vi "Example-AI Scope IN+Signal Processing+AO Wavegen OUT.vi"() -> ()   [LabVIEW 2018]
uses:
  <vilib>/Analysis/3filter.llb/Filter Passband Type.ctl
  <vilib>/Analysis/NI_AALBase.lvlib
  <vilib>/Analysis/3filter.llb/Butterworth Filter (DBL).vi
panel:
  out "Description":string
  out "SerialNumber":string
  out "return":i32
  in  "timeout":i32=1
  in  "delay(ms)":i32=10
  in  "Getscope":bool
  in  "Filter Config 2":T2={"filter type"=enum."Lowpass", "sampling freq: fs"=800000.0, "high cutoff freq: fh"=10000000.0, "low cutoff freq: fl"=100000.0, "order"=2} {"sampling freq: fs" format="%0.2f"; "high cutoff freq: fh" format="%0.2f"; "low cutoff freq: fl" format="%0.4f"}
  in  "Filter Config":T2={"filter type"=enum."Lowpass", "sampling freq: fs"=800000.0, "high cutoff freq: fh"=10000000.0, "low cutoff freq: fl"=1000.0, "order"=2} {"sampling freq: fs" format="%0.2f"; "high cutoff freq: fh" format="%0.2f"; "low cutoff freq: fl" format="%0.4f"}
  in  "停止":bool
  in  "CH2":T3={"ch"=1, "amp"=1.0, "vOffset"=0.0, "hzFrequency"=2000, "percentageSymmetry"=50.0, "degreePhase"=0.0, "func"=enum."Sine"}
  in  "CH1":T3={"ch"=0, "amp"=1.0, "vOffset"=0.0, "hzFrequency"=2000, "percentageSymmetry"=50.0, "degreePhase"=0.0, "func"=enum."Sine"}
  out "Scope Graph":cluster{"voltages":dbl[], "voltages":dbl[]}[](graph) caption="XY图"
  in  "trigcond":enum16{"Raising", "Falling", "Either"}(ring)
  in  "trigsrc":T4(ring)=enum."DetectorAnalogInCH1"
  in  "trigtype":enum16{"edge", "pulse", "trasition"}(ring)
  in  "enable 2":bool=TRUE
  in  "range 2":dbl=5.0
  in  "voltsLevel":dbl
  in  "range":dbl=5.0
  in  "enable":bool=TRUE
  in  "buffersize":i32=2048
  out "Scope returns":i32[](array[numeric])
  in  "fre":i32=800000
  out "error out":errorcluster caption="错误输出"
  out "ftHandle out":u64=372147880
  in  "Device Index":i32
  # "Scope Config"
  # "Function Wave Generation"
  # "Filter"
  # "Tips: CH1 Filter fl < Wavegen Frequency"
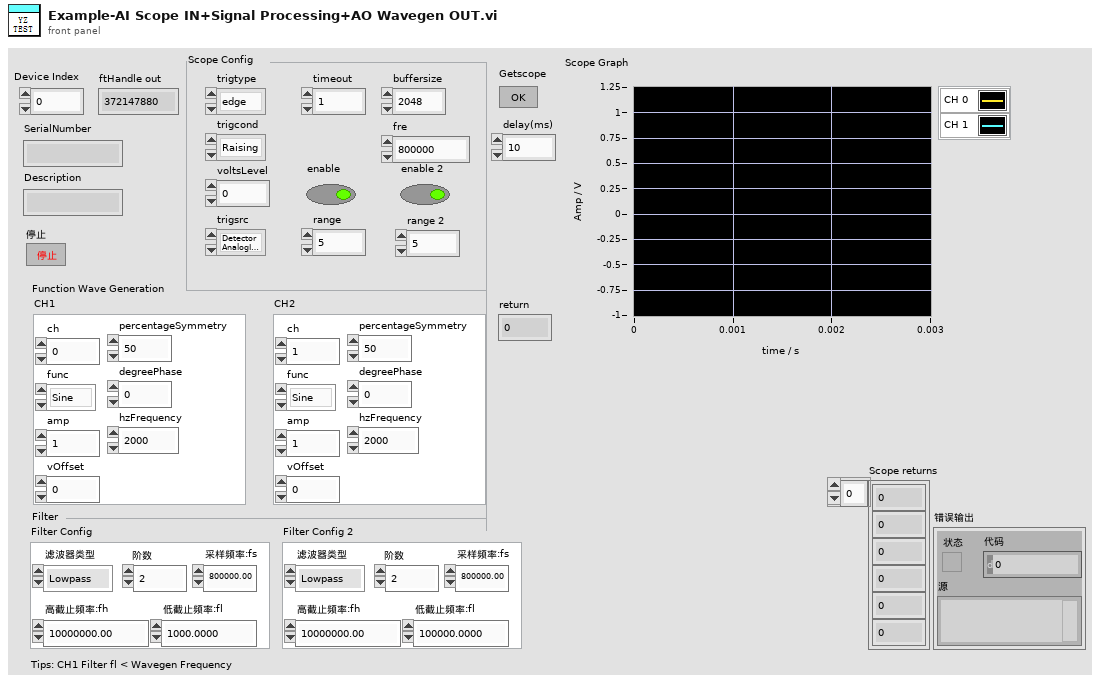
[diagram p1: front panel]
types:
  T1 = typedef "NI_AALBase.lvlib/Filter Passband Type.ctl" = enum32{"Lowpass", "Highpass", "Bandpass", "Bandstop"}
  T2 = cluster{"filter type":T1, "sampling freq: fs":dbl, "high cutoff freq: fh":dbl, "low cutoff freq: fl":dbl, "order":i32}
  T3 = cluster{"ch":i32, "amp":dbl, "vOffset":dbl, "hzFrequency":i32, "percentageSymmetry":dbl, "degreePhase":dbl, "func":enum8{"DC", "Sine", "Square", "Triangle", "RampUp", "RampDown", "Noise", "Pulse", "Trapezium", "SinePower", "Custom", "Play"}}
  T4 = enum16{"None", "DetectorAnalogInCH1", "DetectorAnalogInCH2", "AnalogOut1", "AnalogOut2", "DetectorDigitalIn", "DigitalOut", "Manule", "External 1", "External 2", "DigitalIn"}
  T5 = enum16{"CLIFFStateReady", "CLIFFStateArmed", "CLIFFStateDone", "CLIFFStateRunning", "CLIFFStateConfig", "CLIFFStatePrefill", "CLIFFStateTriggered", "CLIFFStateWait"}
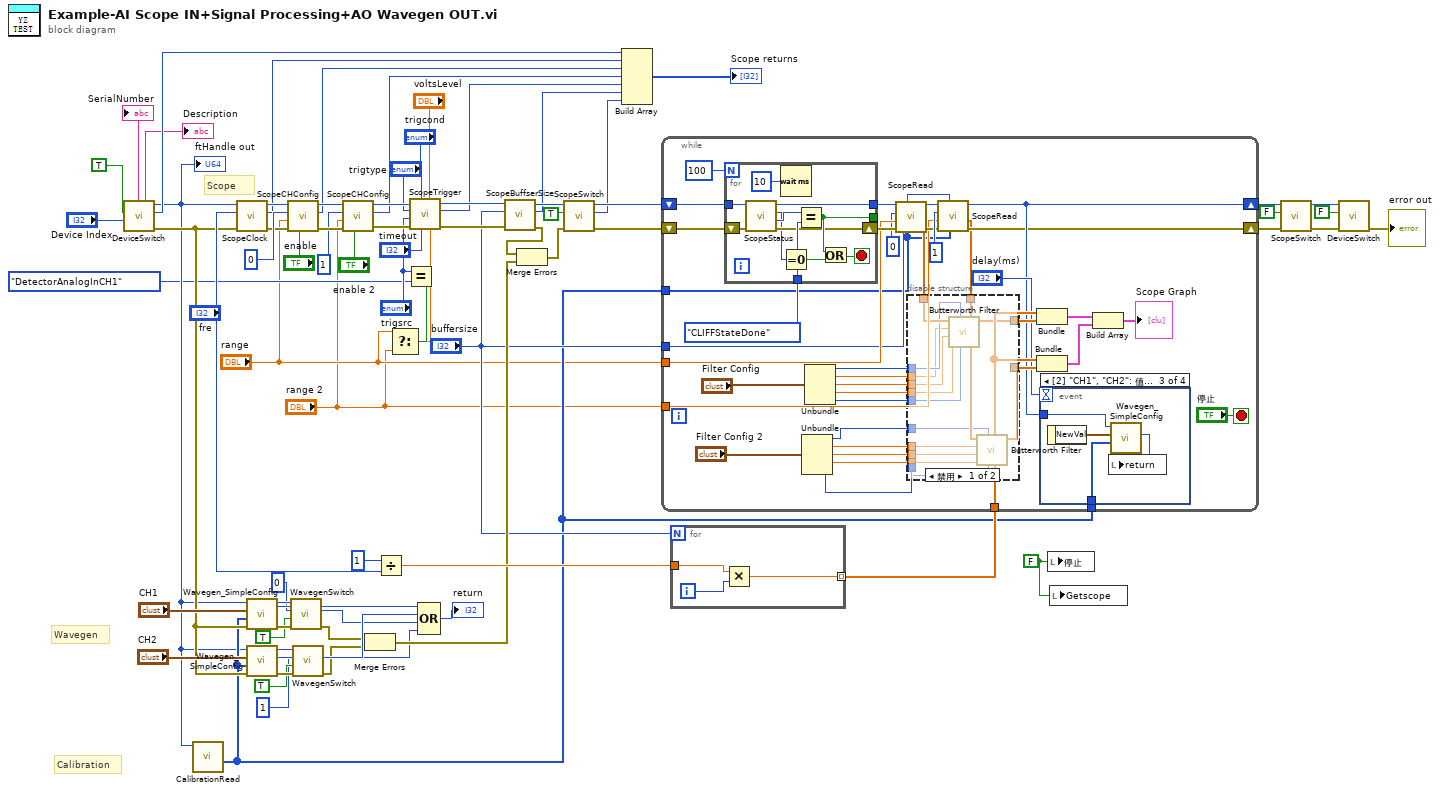
[diagram p0: block diagram]
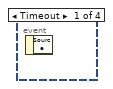
[diagram p2: hidden frame]
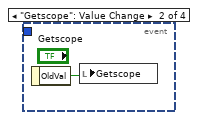
[diagram p3: hidden frame]
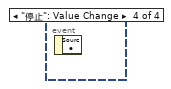
[diagram p4: hidden frame]
diagram:
  w69 = FALSE ("停止")
  # "Scope"
  # "Wavegen"
  # "Calibration"
  n1 = call "DeviceSwitch.vi"("Device Index"="Device Index", "Open"=TRUE) -> ("error out"=w27:errorcluster, "function return"=w38:i32, "handle out"=w7:u64, "Description"=→"Description":string, "SerialNumber"=→"SerialNumber":string)  [unwired: 5 in]
  "ftHandle out" <- w7
  n2 = call "CalibrationRead.vi"("handle"=w7) -> ("CalArray"=w8:u8[])  [unwired: 6 in, 3 out]
  n3 = call "ScopeClock.vi"("error in (no error)"=w27, "fre(Hz)"="fre", "handle"=w7) -> ("error out"=w61:errorcluster, "function return"=w36:i32, "handle out"=w63:u64)  [unwired: 6 in]
  n4 = call "Wavegen_SimpleConfig.vi"("error in (no error)"=w27, "CalArray"=w8, "参数"="CH1", "ftHandle"=w7) -> ("error out"=w18:errorcluster, "function out"=w26:i32, "ftHandle out"=w15:u64)  [unwired: 5 in]
  n5 = call "Wavegen_SimpleConfig.vi"("error in (no error)"=w27, "CalArray"=w8, "参数"="CH2", "ftHandle"=w7) -> ("error out"=w21:errorcluster, "function out"=w25:i32, "ftHandle out"=w14:u64)  [unwired: 5 in]
  n6 = call "ScopeCHConfig.vi"("enable"="enable", "error in (no error)"=w61, "range(V)"="range", "CH"=0 ("channel 3"), "handle"=w63) -> ("error out"=w65:errorcluster, "function return"=w35:i32, "handle out"=w64:u64)  [unwired: 4 in]
  n7 = call "WavegenSwitch.vi"("error in (no error)"=w18, "output"=TRUE, "ch"=0, "ftHandle"=w15) -> ("error out"=w19:errorcluster, "function out"=w13:i32)  [unwired: 5 in, 1 out]
  n8 = call "WavegenSwitch.vi"("error in (no error)"=w21, "output"=TRUE, "ch"=1, "ftHandle"=w14) -> ("error out"=w20:errorcluster, "function out"=w12:i32)  [unwired: 5 in, 1 out]
  n9 = call "ScopeCHConfig.vi"("enable"="enable 2", "error in (no error)"=w65, "range(V)"="range 2", "CH"=1 ("channel 2"), "handle"=w64) -> ("error out"=w58:errorcluster, "function return"=w34:i32, "handle out"=w59:u64)  [unwired: 4 in]
  n10 = Merge Errors(w19, w20) -> (w70:errorcluster)
  n11 = Divide(x=1, y="fre") -> (x/y=w72:dbl)
  n12 = Equal?(x="trigsrc", y=T4."DetectorAnalogInCH1") -> (x = y?=w4:bool)
  n13 = Select(t="range", s=w4, f="range 2") -> (s? t:f=w1:dbl)
  n14 = call "ScopeTrigger.vi"("range"=w1, "voltsLevel"="voltsLevel", "timeout"="timeout", "trigcond"="trigcond", "error in (no error)"=w58, "trigsrc"="trigsrc", "trigtype"="trigtype", "handle"=w59) -> ("error out"=w52:errorcluster, "function return"=w33:i32, "handle out"=w51:u64)  [unwired: 1 in]
  n15 = Compound Arithmetic op=OR ("复合运算")(w26, w25, w13, w12) -> (→"return":i32)
  n16 = call "ScopeBuffserSize.vi"("error in (no error)"=w52, "BufferSize"="buffersize", "handle"=w51) -> ("error out"=w49:errorcluster, "function return"=w32:i32, "handle out"=w47:u64)  [unwired: 6 in]
  n17 = Merge Errors(w49, w70) -> (w48:errorcluster)
  n18 = call "ScopeSwitch.vi"("error in (no error)"=w48, "Run"=TRUE ("run"), "handle"=w47) -> ("error out"=w44:errorcluster, "function return"=w31:i32, "handle out"=w45:u64)  [unwired: 6 in]
  n19 = Build Array(w38, w36, w35, w34, w33, w32, w31) -> (→"Scope returns":i32[])
  n20 = for {
    N: "buffersize" -> [_]
    tunnel: w72 -> [w76]
    tunnel: [w75] -> w71 mode=indexing
    i -> [w77]
    n21 = Multiply(x=w76, y=w77) -> (x*y=w75:dbl)
  }
  n22 = while {
    tunnel: "range" -> [w90]
    tunnel: "range 2" -> [w87]
    tunnel: "buffersize" -> [w80]
    tunnel: w71 -> [w109]
    shift-right: [w85] -> w43
    shift-left: w45 -> [w116]
    shift-right: [w84] -> w40
    shift-left: w44 -> [w115]
    tunnel: w8 -> [w79]
    tunnel: w8 -> [w78]
    stop <- "停止" stop-if-true
    n23 = for {
      N: 100 -> [_]
      tunnel: w116 -> [w142]
      shift-right: [w140] -> w91
      shift-left: w115 -> [w143]
      tunnel: T5."CLIFFStateDone" ("ANIStatus") -> [w148]
      tunnel: [w141] -> w92
      tunnel: [w147] -> _
      stop <- w145 stop-if-true
      n24 = call "ScopeStatus.vi"("error in (no error)"=w143, "handle"=w142) -> ("error out"=w140:errorcluster, "ANIStatus"=w139:T5, "function return"=w138:i32, "handle out"=w141:u64)  [unwired: 6 in]
      n25 = Wait (ms)(milliseconds to wait=u32 10 ("等待时间（毫秒）")) -> ()  [unwired: 1 out]
      n26 = Equal To 0?(x=w138) -> (x = 0?=w144:bool)
      n27 = Equal?(x=w139, y=w148) -> (x = y?=w147:bool)
      n28 = Or(x=w147, y=w144) -> (x .or. y?=w145:bool)
    }
    n29 = Unbundle("Filter Config 2") -> ("filter type"=w94:T1, "sampling freq: fs"=w98:dbl, "high cutoff freq: fh"=w97:dbl, "low cutoff freq: fl"=w96:dbl, "order"=w95:i32)
    n30 = Unbundle("Filter Config") -> ("filter type"=w105:T1, "sampling freq: fs"=w104:dbl, "high cutoff freq: fh"=w103:dbl, "low cutoff freq: fl"=w102:dbl, "order"=w101:i32)
    n31 = call "ScopeRead.vi"("CalArray"=w79, "BufferSize"=w80, "error in (no error)"=w91, "Range"=w90, "ch"=0, "handle"=w92) -> ("error out"=w88:errorcluster, "voltages"=w83:dbl[], "handle out"=w86:u64)  [unwired: 1 in, 2 out]
    n32 = call "ScopeRead.vi"("CalArray"=w79, "BufferSize"=w80, "error in (no error)"=w88, "Range"=w87, "ch"=1, "handle"=w86) -> ("error out"=w84:errorcluster, "voltages"=w82:dbl[], "handle out"=w85:u64)  [unwired: 1 in, 2 out]
    n33 = disable-structure shown="禁用" {
      disable-tunnel: w83 -> [w135 w136]
      disable-tunnel: [w134 w136] -> w107
      disable-tunnel: w105 -> [w133 _]
      disable-tunnel: w104 -> [w132 _]
      disable-tunnel: w103 -> [w131 _]
      disable-tunnel: w102 -> [w130 _]
      disable-tunnel: w101 -> [w129 _]
      disable-tunnel: [w128 w137] -> w99
      disable-tunnel: w82 -> [w127 w137]
      disable-tunnel: w98 -> [w126 _]
      disable-tunnel: w97 -> [w125 _]
      disable-tunnel: w96 -> [w124 _]
      disable-tunnel: w95 -> [w123 _]
      disable-tunnel: w94 -> [w122 _]
      frame Disabled {
        n34 = call-poly <vilib>:"Butterworth Filter.vi"("order"=w129, "filter type"=w133, "low cutoff freq: fl"=w130, "high cutoff freq: fh"=w131, "sampling freq: fs"=w132, "X"=w135) -> ("Filtered X"=w134:dbl[])  [unwired: 2 in, 1 out]
        n35 = call-poly <vilib>:"Butterworth Filter.vi"("order"=w123, "filter type"=w122, "low cutoff freq: fl"=w124, "high cutoff freq: fh"=w125, "sampling freq: fs"=w126, "X"=w127) -> ("Filtered X"=w128:dbl[])  [unwired: 2 in, 1 out]
      }
      frame Enabled {
      }
    }
    n36 = Bundle(w109, "voltages"=w107) -> (w112:cluster{dbl[], "voltages":dbl[]})  [unwired: 1 in]
    n37 = Bundle(w109, "voltages"=w99) -> (w111:cluster{dbl[], "voltages":dbl[]})  [unwired: 1 in]
    n38 = event shown="[2] \"CH1\", \"CH2\": 值改变" {
      selector: _ -> [_ _ _ _]
      dyn-events: _ -> [_ _ _ _]
      timeout: "delay(ms)" -> [_ _ _ _]
      tunnel: w85 -> [_ _ w121 _]
      tunnel: w78 -> [_ _ w118 _]
      event Timeout {
        n39 = event-data() -> ()  [unwired: 1 in, 1 out]
      }
      event "Getscope": Value Change {
        n40 = event-data() -> ("OldVal"=w117:bool)  [unwired: 1 in]
        n41 = local write "Getscope"(w117) -> ()
      }
      event "CH1", "CH2": Value Change {
        n42 = event-data() -> ("NewVal"=w120:T3)  [unwired: 1 in]
        n43 = call "Wavegen_SimpleConfig.vi"("CalArray"=w118, "参数"=w120, "ftHandle"=w121) -> ("function out"=w119:i32)  [unwired: 6 in, 2 out]
        n44 = local write "return"(w119) -> ()
      }
      event "停止": Value Change {
        n45 = event-data() -> ()  [unwired: 1 in, 1 out]
      }
    }
    n46 = Build Array(w112, w111) -> (→"Scope Graph":cluster{dbl[], "voltages":dbl[]}[])
  }
  n47 = local write "停止"(w69) -> ()
  n48 = local write "Getscope"(w69) -> ()
  n49 = call "ScopeSwitch.vi"("error in (no error)"=w40, "Run"=FALSE, "handle"=w43) -> ("error out"=w41:errorcluster, "handle out"=w42:u64)  [unwired: 6 in, 1 out]
  n50 = call "DeviceSwitch.vi"("error in (no error)"=w41, "Open"=FALSE, "handle"=w42) -> ("error out"=→"error out":errorcluster)  [unwired: 4 in, 4 out]
